vi "IMAQ FPGA CXP Data to Vision Pixel Bus 8-Bit x 32.vi"(7 "Reset":bool, 10 "Image Size":cluster{"Width":u16, "Height":u16}, 11 "CXP Data":T1) -> (0 "EOI":bool, 1 "EOL":bool, 2 "DV":bool[](array[boolean]), 3 "Pixel Data":u8[](array[numeric]), 4 "Ready for Input":bool)   [LabVIEW 2020]
uses:
  <vilib>/visionFPGA/Basics/CoaXPress Acquisition/Controls/IMAQ FPGA CXP NI AXI4-S Bus.ctl
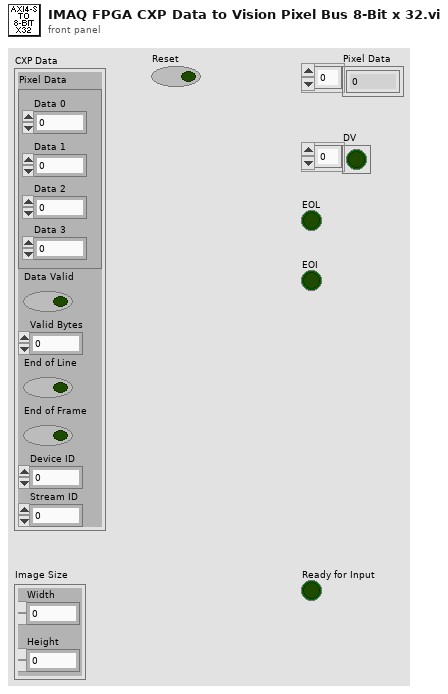
[diagram p1: front panel]
types:
  T1 = typedef "IMAQ FPGA CXP NI AXI4-S Bus.ctl" = cluster{"Pixel Data":cluster{"Data 0":u64, "Data 1":u64, "Data 2":u64, "Data 3":u64}, "Data Valid":bool, "Valid Bytes":u8, "End of Line":bool, "End of Frame":bool, "Device ID":u8, "Stream ID":u8}
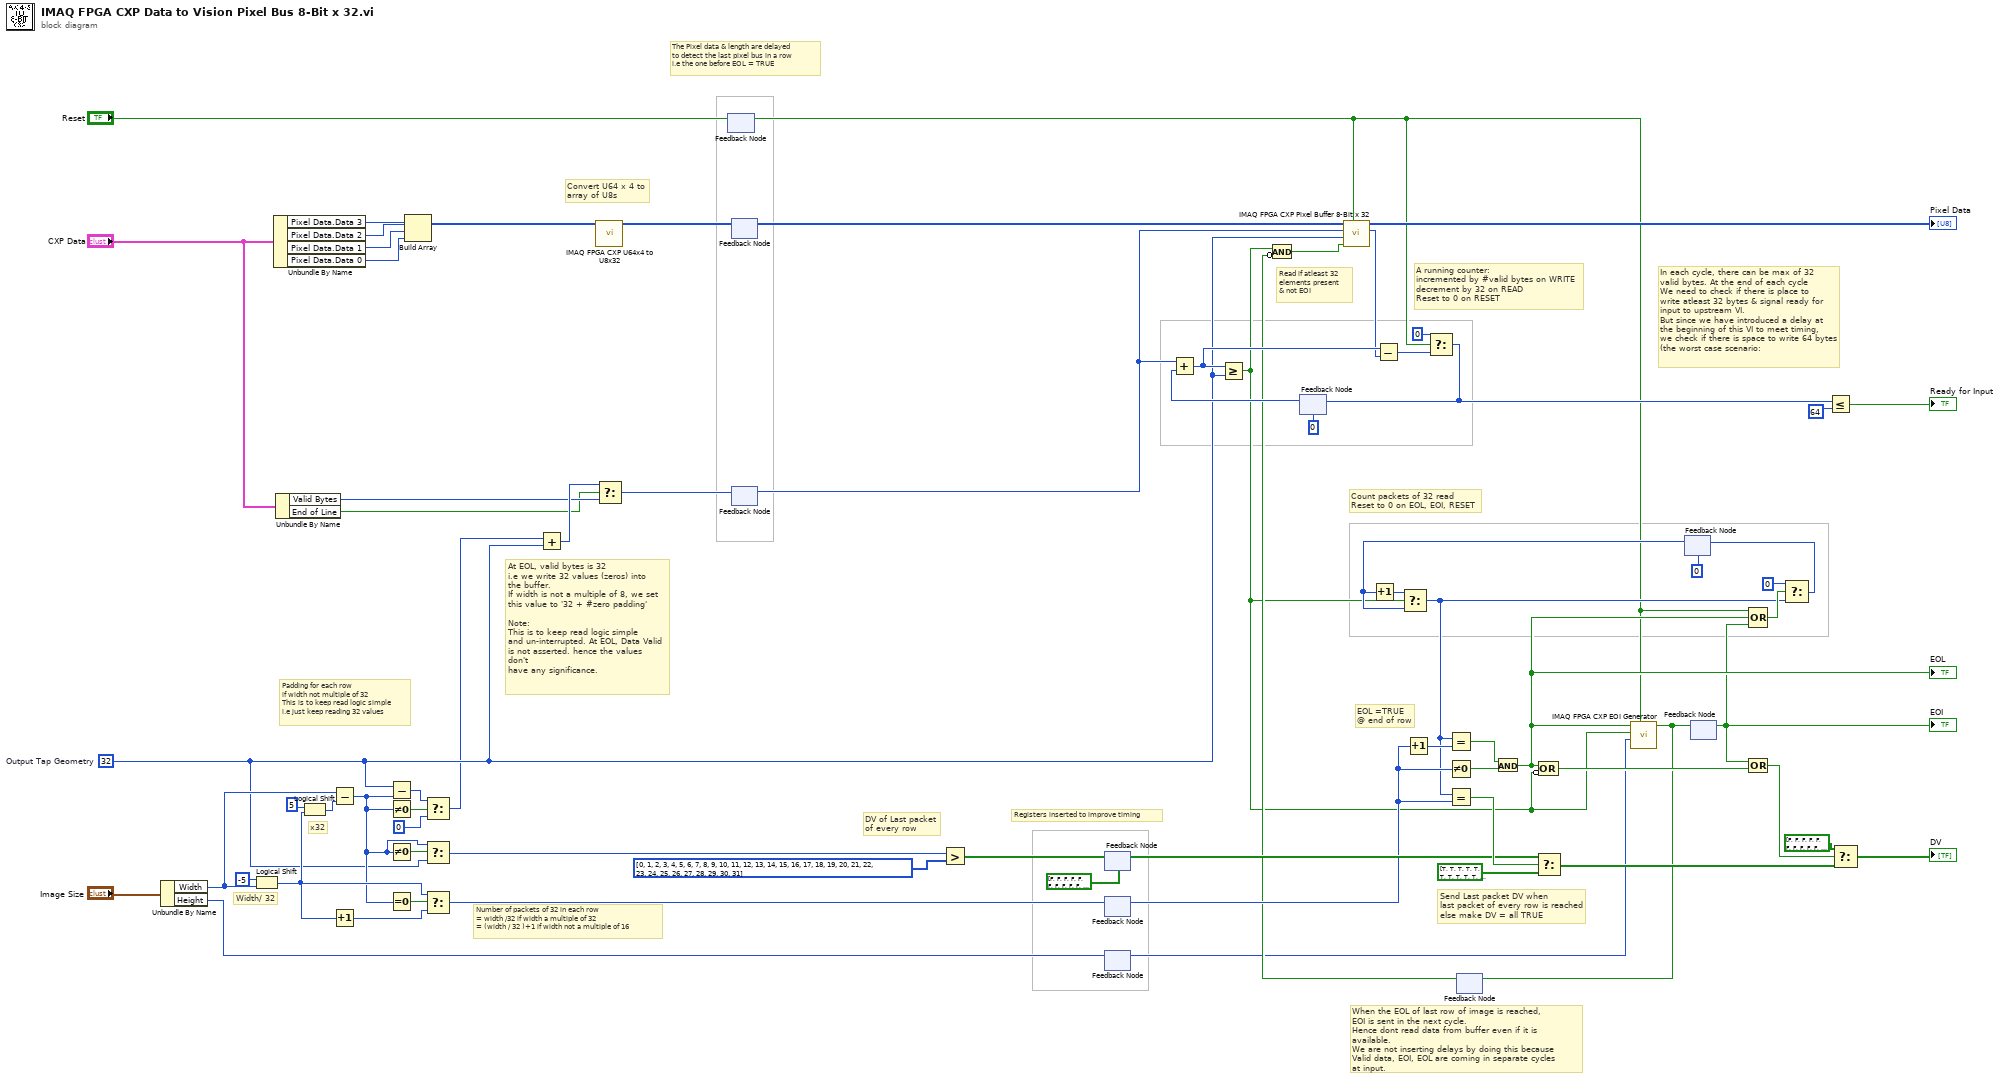
[diagram p0: block diagram]
diagram:
  w17 = u8 32  # Output Tap Geometry
  # "Padding for each row\nif width not multiple of 32\nThis is to keep read logic simple\ni.e just keep reading 32 values"
  # "x32"
  # "Width/ 32"
  # "When the EOL of last row of image is reached,\nEOI is sent in the next cycle. \nHence dont read data from buffer even if it is available.\nWe are not inserting delays by doing this because \nValid data, EOI, EOL are coming in separate cycles\nat input."
  # "EOL =TRUE\n@ end of row"
  # "Count packets of 32 read\nReset to 0 on EOL, EOI, RESET"
  # "Send Last packet DV when\nlast packet of every row is reached\nelse make DV = all TRUE"
  # "A running counter:\nincremented by #valid bytes on WRITE\ndecrement by 32 on READ\nReset to 0 on RESET"
  # "Convert U64 x 4 to \narray of U8s"
  # "In each cycle, there can be max of 32\nvalid bytes. At the end of each cycle\nWe need to check if there is place to \nwrite atleast 32 bytes & signal ready for\ninput to upstream VI.\nBut since we have introduced a delay at\nthe beginning of this VI to meet timing,\nwe check if there is space to write 64 bytes\n(the worst case scenario:"
  # "Read if atleast 32\nelements present\n& not EOI"
  # "Number of packets of 32 in each row\n= width /32 if width a multiple of 32\n= (width / 32 )+1 if width not a multiple of 16"
  # "DV of Last packet \nof every row"
  # "At EOL, valid bytes is 32\ni.e we write 32 values (zeros) into\nthe buffer.\nIf width is not a multiple of 8, we set\nthis value to '32 + #zero padding'\n\nNote:\nThis is to keep read logic simple\nand un-interrupted. At EOL, Data Valid\nis not asserted. hence the values don't\nhave any significance."
  # "Registers inserted to improve timing"
  # "The Pixel data & length are delayed\nto detect the last pixel bus in a row\ni.e the one before EOL = TRUE"
  n1 = Unbundle By Name("Image Size") -> ("Width"=w42:u16, "Height"=w35:u16)
  n2 = Logical Shift(y=i16 -5, x=w42) -> (x << y=w52:u16)
  n3 = Unbundle By Name("CXP Data") -> ("Pixel Data.Data 3"=w24:u64, "Pixel Data.Data 2"=w23:u64, "Pixel Data.Data 1"=w22:u64, "Pixel Data.Data 0"=w21:u64)
  n4 = Unbundle By Name("CXP Data") -> ("Valid Bytes"=w25:u8, "End of Line"=w7:bool)
  n5 = Logical Shift(y=i16 5, x=w52) -> (x << y=w48:u16)
  n6 = Subtract(x=w42, y=w48) -> (x-y=w46:u16)
  n7 = Increment(x=w52) -> (x+1=w64:u16)
  n8 = Subtract(x=w17, y=w46) -> (x-y=w49:u8)
  n9 = Not Equal To 0?(x=w46) -> (x != 0?=w50:bool)
  n10 = Not Equal To 0?(x=w46) -> (x != 0?=w47:bool)
  n11 = Equal To 0?(x=w46) -> (x = 0?=w65:bool)
  n12 = Build Array(w24, w23, w22, w21) -> (w57:u64[])
  n13 = Select(t=w49, s=w50, f=u8 0 ("x")) -> (s? t:f=w15:u8)
  n14 = Select(t=w46, s=w47, f=w17) -> (s? t:f=w45:u16)
  n15 = Select(t=w52, s=w65, f=w64) -> (s? t:f=w36:u16)
  n16 = Add(x=w15, y=w17) -> (x+y=w31:u8)
  n17 = call <vilib>:"IMAQ FPGA CXP U64x4 to U8x32.vi"("Pixel Data U64x4"=w57) -> ("Pixel Data Out U8x32"=w27:u8[])  [unwired: 10 in]
  n18 = Select(t=w31, s=w7, f=w25) -> (s? t:f=w56:u8)
  n19 = feedback-in #1("Reset") -> ()
  n20 = feedback #1() -> (w1:bool)  [unwired: 1 in]
  n21 = feedback-in #2(w27) -> ()
  n22 = feedback #2() -> (w9:u8[])  [unwired: 1 in]
  n23 = feedback-in #3(w56) -> ()
  n24 = feedback #3() -> (w10:u8)  [unwired: 1 in]
  n25 = Greater?(x=w45, y=u16[] [0, 1, 2, 3, 4, 5, 6, 7, 8, 9, 10, 11, 12, 13, 14, 15, 16, 17, 18, 19, 20, 21, 22, 23, 24, 25, 26, 27, 28, 29, 30, 31]) -> (0:w38:bool[])
  n26 = feedback #4(bool[] [FALSE, FALSE, FALSE, FALSE, FALSE, FALSE, FALSE, FALSE, FALSE, FALSE, FALSE, FALSE, FALSE, FALSE, FALSE, FALSE, FALSE, FALSE, FALSE, FALSE, FALSE, FALSE, FALSE, FALSE, FALSE, FALSE, FALSE, FALSE, FALSE, FALSE, FALSE, FALSE] ("x > y?")) -> (w37:bool[])
  n27 = feedback-in #4(w38) -> ()
  n28 = feedback #5() -> (w29:u16)  [unwired: 1 in]
  n29 = feedback-in #5(w36) -> ()
  n30 = feedback #6() -> (w4:u16)  [unwired: 1 in]
  n31 = feedback-in #6(w35) -> ()
  n32 = feedback #7(u8 0) -> (w71:u8)
  n33 = Add(x=w10, y=w71) -> (x+y=w70:u8)
  n34 = Greater Or Equal?(x=w70, y=w17) -> (x >= y?=w5:bool)
  n35 = Increment(x=w29) -> (x+1=w30:u16)
  n36 = Not Equal To 0?(x=w29) -> (x != 0?=w32:bool)
  n37 = feedback #8() -> (w16:bool)  [unwired: 1 in]
  n38 = Compound Arithmetic op=AND(w5, invert w16) -> (w11:bool)
  n39 = call <vilib>:"IMAQ FPGA CXP Pixel Buffer 8-Bit x 32.vi"("Reset"=w1, "Read"=w11, "Tap"=w17, "Valid Bytes"=w10, "Pixel Data In U8x32"=w9) -> ("#Elements Read"=w18:u8, "Pixel Data Out U8x8"=→"Pixel Data":u8[])  [unwired: 5 in]
  n40 = Subtract(x=w70, y=w18) -> (x-y=w13:u8)
  n41 = Select(t=u8 0, s=w1, f=w13) -> (s? t:f=w12:u8)
  n42 = feedback-in #7(w12) -> ()
  n43 = feedback #9(u16 0) -> (w44:u16)
  n44 = Increment(x=w44) -> (x+1=w62:u16)
  n45 = Select(t=w62, s=w5, f=w44) -> (s? t:f=w28:u16)
  n46 = Equal?(x=w28, y=w30) -> (x = y?=w33:bool)
  n47 = Equal?(x=w28, y=w29) -> (x = y?=w61:bool)
  n48 = And(x=w33, y=w32) -> (x .and. y?=w6:bool)
  "EOL" <- w6
  n49 = Select(t=w37, s=w61, f=bool[] [TRUE, TRUE, TRUE, TRUE, TRUE, TRUE, TRUE, TRUE, TRUE, TRUE, TRUE, TRUE, TRUE, TRUE, TRUE, TRUE, TRUE, TRUE, TRUE, TRUE, TRUE, TRUE, TRUE, TRUE, TRUE, TRUE, TRUE, TRUE, TRUE, TRUE, TRUE, TRUE] ("x > y?")) -> (s? t:f=w59:bool[])
  n50 = Compound Arithmetic op=OR(w6, invert w5) -> (w41:bool)
  n51 = call <vilib>:"IMAQ FPGA CXP EOI Generator.vi"("Reset"=w1, "Height"=w4, "Enable"=w5, "EOL"=w6) -> ("EOI"=w3:bool)  [unwired: 7 in]
  n52 = feedback-in #8(w3) -> ()
  n53 = feedback-in #10(w3) -> ()
  n54 = feedback #10() -> (w2:bool)  [unwired: 1 in]
  "EOI" <- w2
  n55 = Compound Arithmetic op=OR(w1, w6, w2) -> (w39:bool)
  n56 = Compound Arithmetic op=OR(w2, w41) -> (w40:bool)
  n57 = Select(t=u16 0, s=w39, f=w28) -> (s? t:f=w55:u16)
  n58 = feedback-in #9(w55) -> ()
  n59 = Less Or Equal?(x=w12, y=u8 64) -> (x <= y?=→"Ready for Input":bool)
  n60 = Select(t=bool[] [FALSE, FALSE, FALSE, FALSE, FALSE, FALSE, FALSE, FALSE, FALSE, FALSE, FALSE, FALSE, FALSE, FALSE, FALSE, FALSE, FALSE, FALSE, FALSE, FALSE, FALSE, FALSE, FALSE, FALSE, FALSE, FALSE, FALSE, FALSE, FALSE, FALSE, FALSE, FALSE] ("x > y?"), s=w40, f=w59) -> (s? t:f=→"DV":bool[])
